vi "Test new input configeration.vi"() -> ()   [LabVIEW 2024]
uses:
  C:/Users/CHEM-2XN7PR3/Desktop/Testing/Monoterm/MonoTerm 5.1 Source/Mono Term/DLL/Cornerstone.dll
  Monoterm/MonoTerm 5.1 Source/Mono Term/DLL/Cornerstone.dll
  Monoterm/MonoTerm 5.1 Source/Mono Term/Typedefs/USBCornerstone deviceID.ctl
panel:
  out "string":string
  out "Variant Out":variant
  out "error out":errorcluster
  in  "error in (no error)":errorcluster
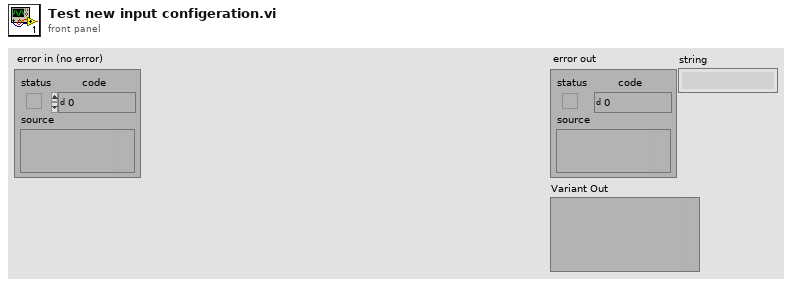
[diagram p1: front panel]
types:
  T1 = typedef "USBCornerstone deviceID.ctl" = i32
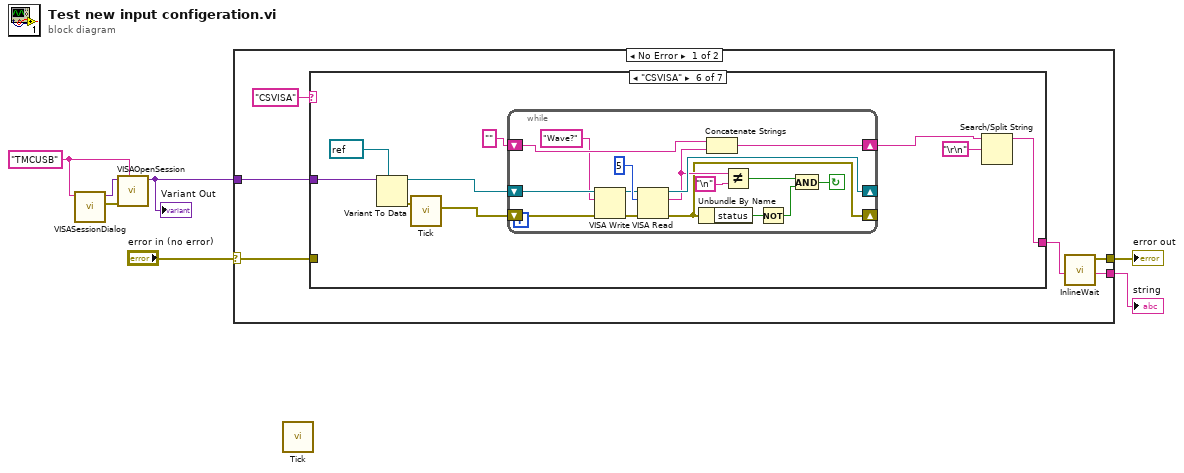
[diagram p0: block diagram]
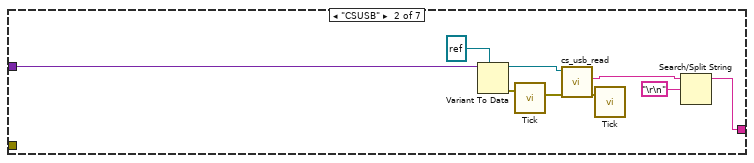
[diagram p3: hidden frame]
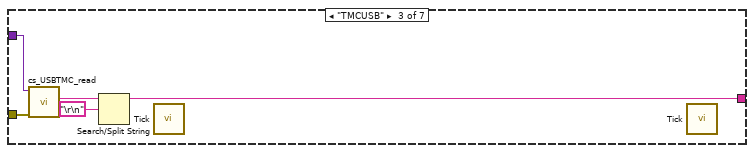
[diagram p4: hidden frame]
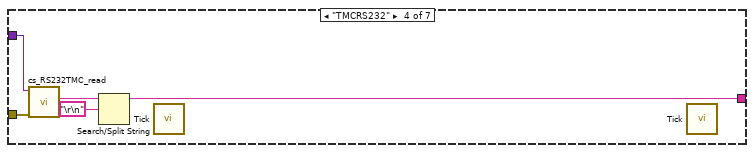
[diagram p5: hidden frame]
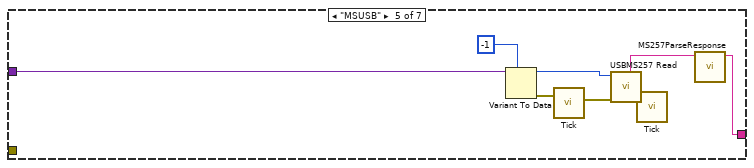
[diagram p6: hidden frame]
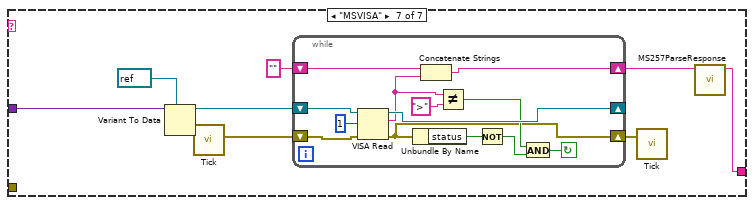
[diagram p7: hidden frame]
diagram:
  w2 = "TMCUSB" ("Resource Type")
  n1 = call "VISASessionDialog.vi"("Resource Type"=w2) -> ("Error Out"=w4:errorcluster, "Variant"=w3:variant)  [unwired: 9 in]
  n2 = call "VISAOpenSession.vi"("Resource Type"=w2, "error in (no error)"=w4, "Variant"=w3) -> ("Variant Out"=w1:variant)  [unwired: 7 in, 1 out]
  "Variant Out" <- w1
  n3 = case shown="No Error" "error in (no error)" {
    selector: "error in (no error)" -> [w9 w87]
    tunnel: w1 -> [w12 _]
    tunnel: [w11 w87] -> w6
    tunnel: [w10 _] -> w5
    frame No Error {
      n4 = case shown="\"CSVISA\"" "CSVISA" {
        tunnel: w12 -> [_ w20 w24 w29 w39 w48 w73]
        tunnel: [_ w16 w25 w30 w36 w42 w68] -> w10
        tunnel: w9 -> [_ _ w23 w28 _ _ _]
        frame "None", Default {
        }
        frame "CSUSB" {
          n5 = Variant To Data(type=refnum<k24> refnum ("reference out"), Variant=w20) -> (data=w19:refnum<k24>, error out=w15:errorcluster)  [unwired: 1 in]
          n6 = call "Tick.vi"("Error In"=w15) -> ("Error Out"=w14:errorcluster)  [unwired: 9 in, 1 out]
          n7 = call "cs_usb_read.vi"("error in (no error)"=w14, "new reference"=w19) -> ("error out"=w13:errorcluster, "string"=w17:string)  [unwired: 7 in, 1 out]
          n8 = call "Tick.vi"("Error In"=w13) -> ()  [unwired: 9 in, 2 out]
          n9 = Search/Split String(string=w17, search string/char (-)="\r\n") -> (substring before match=w16:string)  [unwired: 1 in, 2 out]
        }
        frame "TMCUSB" {
          n10 = call "cs_USBTMC_read.vi"("error in (no error)"=w23, "Variant In"=w24) -> ("string"=w22:string)  [unwired: 7 in, 2 out]
          n11 = Search/Split String(string=w22, search string/char (-)="\r\n") -> (substring before match=w25:string)  [unwired: 1 in, 2 out]
          n12 = call "Tick.vi"() -> ()  [unwired: 10 in, 2 out]
          n13 = call "Tick.vi"() -> ()  [unwired: 10 in, 2 out]
        }
        frame "TMCRS232" {
          n14 = call "cs_RS232TMC_read.vi"("error in (no error)"=w28, "Variant In"=w29) -> ("string"=w27:string)  [unwired: 7 in, 2 out]
          n15 = Search/Split String(string=w27, search string/char (-)="\r\n") -> (substring before match=w30:string)  [unwired: 1 in, 2 out]
          n16 = call "Tick.vi"() -> ()  [unwired: 10 in, 2 out]
          n17 = call "Tick.vi"() -> ()  [unwired: 10 in, 2 out]
        }
        frame "MSUSB" {
          n18 = Variant To Data(type=T1 -1 ("cs_deviceID"), Variant=w39) -> (data=w37:T1, error out=w34:errorcluster)  [unwired: 1 in]
          n19 = call "Tick.vi"("Error In"=w34) -> ("Error Out"=w32:errorcluster)  [unwired: 9 in, 1 out]
          n20 = call "USBMS257 Read.vi"("error in (no error)"=w32, "cs_deviceID"=w37) -> ("error out"=w33:errorcluster, "response"=w35:string)  [unwired: 5 in, 1 out]
          n21 = call "Tick.vi"("Error In"=w33) -> ()  [unwired: 9 in, 2 out]
          n22 = call "MS257ParseResponse.vi"("response in"=w35) -> ("response out"=w36:string)  [unwired: 10 in]
        }
        frame "CSVISA" {
          n23 = Variant To Data(type=refnum<visa-resource-name> refnum ("VISA resource name"), Variant=w48) -> (data=w45:refnum<visa-resource-name>, error out=w40:errorcluster)  [unwired: 1 in]
          n24 = call "Tick.vi"("Error In"=w40) -> ("Error Out"=w41:errorcluster)  [unwired: 9 in, 1 out]
          n25 = while {
            shift-left: "" -> [w62]
            shift-right: [w63] -> w43
            shift-right: [w60] -> _
            shift-left: w45 -> [w53]
            shift-right: [w54] -> _
            shift-left: w41 -> [w49]
            stop <- w57 continue-if-true
            n26 = VISA Write(VISA resource name=w53, write buffer="Wave?", error in (no error)=w49) -> (VISA resource name out=w52:refnum<visa-resource-name>, error out=w50:errorcluster)  [unwired: 1 out]
            n27 = VISA Read(VISA resource name=w52, byte count=u32 5 ("requested byte count"), error in (no error)=w50) -> (VISA resource name out=w60:refnum<visa-resource-name>, read buffer=w59:string, error out=w54:errorcluster)  [unwired: 1 out]
            n28 = Unbundle By Name(w54) -> ("status"=w58:bool)
            n29 = Concatenate Strings(w62, w59) -> (w63:string)
            n30 = Not Equal?(x=w59, y="\n") -> (x != y?=w55:bool)
            n31 = Not(x=w58) -> (.not. x?=w56:bool)
            n32 = And(x=w55, y=w56) -> (x .and. y?=w57:bool)
          }
          n33 = Search/Split String(string=w43, search string/char (-)="\r\n") -> (substring before match=w42:string)  [unwired: 1 in, 2 out]
        }
        frame "MSVISA" {
          n34 = Variant To Data(type=refnum<visa-resource-name> refnum ("VISA resource name"), Variant=w73) -> (data=w70:refnum<visa-resource-name>, error out=w67:errorcluster)  [unwired: 1 in]
          n35 = call "Tick.vi"("Error In"=w67) -> ("Error Out"=w66:errorcluster)  [unwired: 9 in, 1 out]
          n36 = while {
            shift-left: "" -> [w85]
            shift-right: [w86] -> w69
            shift-right: [w83] -> _
            shift-left: w70 -> [w82]
            shift-right: [w74] -> w65
            shift-left: w66 -> [w81]
            stop <- w75 continue-if-true
            n37 = VISA Read(VISA resource name=w82, byte count=u32 1 ("requested byte count"), error in (no error)=w81) -> (VISA resource name out=w83:refnum<visa-resource-name>, read buffer=w80:string, error out=w74:errorcluster)  [unwired: 1 out]
            n38 = Unbundle By Name(w74) -> ("status"=w77:bool)
            n39 = Concatenate Strings(w85, w80) -> (w86:string)
            n40 = Not Equal?(x=w80, y=">") -> (x != y?=w76:bool)
            n41 = Not(x=w77) -> (.not. x?=w78:bool)
            n42 = And(x=w76, y=w78) -> (x .and. y?=w75:bool)
          }
          n43 = call "Tick.vi"("Error In"=w65) -> ()  [unwired: 9 in, 2 out]
          n44 = call "MS257ParseResponse.vi"("response in"=w69) -> ("response out"=w68:string)  [unwired: 10 in]
        }
      }
      n45 = call "InlineWait.vi"() -> ("Error Out"=w11:errorcluster)  [unwired: 11 in]
    }
    frame Error {
    }
  }
  "error out" <- w6
  "string" <- w5
  n46 = call "Tick.vi"() -> ()  [unwired: 10 in, 2 out]
